vi "Configure SLSC Switch Custom Device.vi"(0 "Target Refnum in":refnum<k24>, 1 "SLSC module":refnum<k21>, 5 "product name":string, 7 "topologies":string[](array[string]), 9 "switches json":string, 11 "error in":errorcluster, 12 "slot number":u32) -> (4 "Target Refnum out":refnum<k24>, 15 "error out":errorcluster)   [LabVIEW 2017, in "SLSC Switch Examples.lvlib"]
uses:
  SLSC Switch Examples.lvlib
  NationalInstruments.VeriStand.SystemDefinitionAPI
  SLSC Switch/Scripting/Properties/SLSC Switch All Properties.ctl
  SLSC Switch/Shared/Endpoint Configuration Cluster.ctl
  SLSC Switch/Shared/Endpoint Configuration Enum.ctl
  SLSC Switch/Scripting/Custom Device/Find SLSC Switch Custom Device by Slot Number.vi
  SLSC Switch/Shared/SLSC Switch Shared.lvlib
  SLSC Switch/Scripting/SLSC Switch Scripting.lvlib
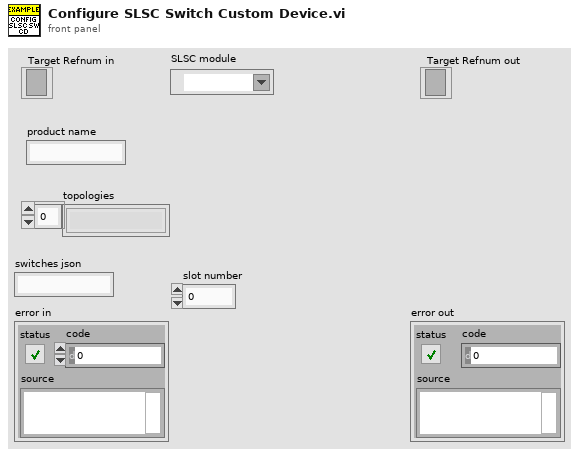
[diagram p1: front panel]
types:
  T1 = typedef "SLSC Switch Scripting.lvlib/SLSC Switch All Properties.ctl" = cluster{"Model":string, "Resource":string, "Topology":string, "Capabilities":string, "Description":string}
  T2 = typedef "Custom Device API.lvlib/Custom Device Item Ref.ctl" = u64
  T3 = typedef "SLSC Switch Shared.lvlib/Endpoint Configuration Enum.ctl" = enum16{"Load", "Source", "Configuration"}
  T4 = typedef "SLSC Switch Shared.lvlib/Endpoint Configuration Cluster.ctl" = cluster{"Endpoint":string, "Configuration":T3}
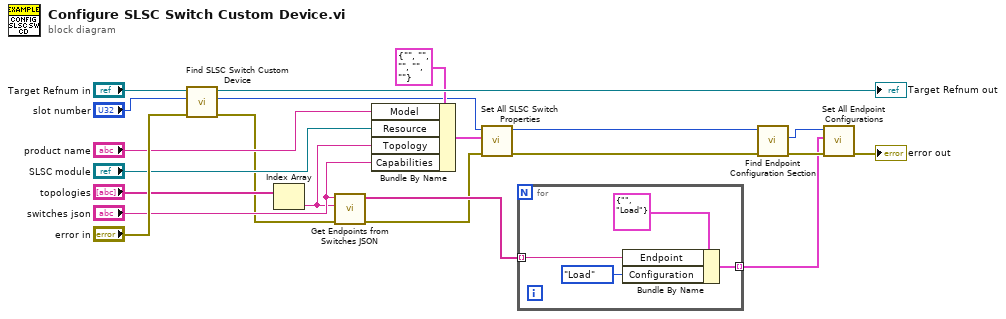
[diagram p0: block diagram]
diagram:
  n1 = call-poly "Find SLSC Switch Custom Device.vi"("error in (no error)"="error in", "slot number"="slot number", "Target in"="Target Refnum in") -> ("error out"=w2:errorcluster, "SLSC Switch Custom Device Ref"=w1:T2, "Target out"=→"Target Refnum out":refnum<k24>)  [unwired: 6 in]
  n2 = Index Array(array="topologies") -> (element=w5:string)  [unwired: 1 in]
  n3 = call "Get Endpoints from Switches JSON.vi"("error in (no error)"=w2, "topology"=w5, "switches json"="switches json") -> ("error out"=w7:errorcluster, "endpoints"=w13:string[])  [unwired: 7 in]
  n4 = Bundle By Name(cluster=T1 {"Model"="", "Resource"="", "Topology"="", "Capabilities"="", "Description"=""} ("SLSC Switch All Properties"), "Model"="product name", "Resource"="SLSC module", "Topology"=w5, "Capabilities"="switches json") -> (w10:T1)
  n5 = call "Set All SLSC Switch Properties.vi"("error in (no error)"=w7, "SLSC Switch All Properties"=w10, "SLSC Switch Custom Device Ref in"=w1) -> ("error out"=w8:errorcluster, "SLSC Switch Custom Device Ref out"=w9:T2)  [unwired: 7 in]
  n6 = for {
    tunnel: w13 -> [w24] mode=indexing
    tunnel: [w22] -> w14 mode=indexing
    n7 = Bundle By Name(cluster=T4 {"Endpoint"="", "Configuration"=enum."Load"} ("All Endpoint Configurations"), "Endpoint"=w24, "Configuration"=Endpoint_Configuration_Enum."Load") -> (w22:T4)
  }
  n8 = call "Find Endpoint Configuration Section.vi"("error in (no error)"=w8, "SLSC Switch Custom Device Ref in"=w9) -> ("error out"=w18:errorcluster, "Endpoint Config Section Ref"=w17:T2)  [unwired: 7 in, 1 out]
  n9 = call "Set All Endpoint Configurations.vi"("error in (no error)"=w18, "All Endpoint Configurations"=w14, "Endpoint Configuration Section Ref in"=w17) -> ("error out"=→"error out":errorcluster)  [unwired: 7 in, 1 out]
